vi "Create Downstream View Cavity Spark Scene.vi"(2 "error in (no error)":errorcluster, 3 "Spark Coordinates (cm, rad, cm)":cluster{"r":sgl, "theta":sgl, "z":sgl}) -> (0 "error out":errorcluster, 1 "reference out":refnum<vi>)   [LabVIEW 2013]
uses:
  <vilib>/Utility/miscctls.llb/LV3DPointTypeDef.ctl
  <vilib>/picture/3D Picture Control/Object/Create Object (name).vi
  <vilib>/picture/3D Picture Control/NI_3D Picture Control.lvlib
panel:
  out "Spark Coordinates (cm, rad, rad)":cluster{"rho":dbl, "theta":dbl, "phi":dbl}
  out "Cavity Upstream View":refnum<vi>(3d-picture)
  out "Spark Coordinates (cm, cm, cm)":T1
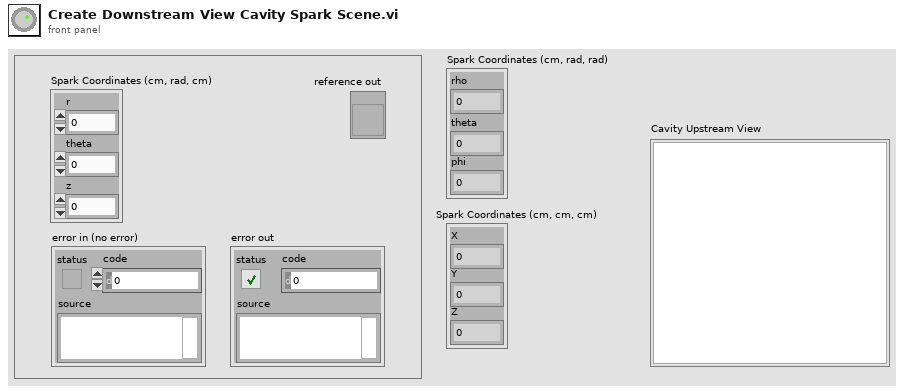
[diagram p1: front panel]
types:
  T1 = typedef "LV3DPointTypeDef.ctl" = cluster{"X":sgl, "Y":sgl, "Z":sgl}
  T2 = cluster{"Red":sgl, "Green":sgl, "Blue":sgl, "Alpha":sgl}
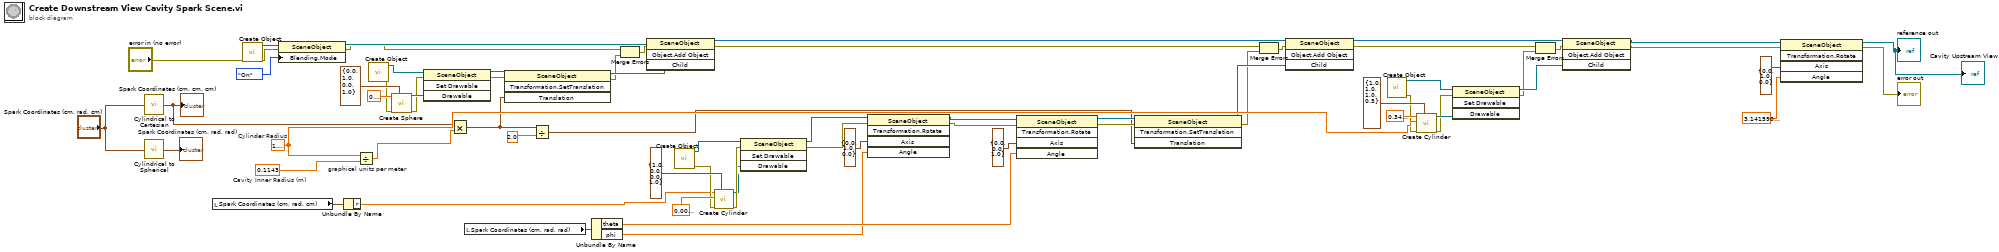
[diagram p0: block diagram]
diagram:
  w52 = 0.1143  # Cavity Inner Radius (m)
  w46 = sgl 1.2  # Cylinder Radius
  n1 = call "Cylindrical to Cartesian.vi"("Cylindrical\nCoordinates"="Spark Coordinates (cm, rad, cm)") -> ("Cartesian\nCoordinates"=w4:cluster{"x":dbl, "y":dbl, "z":dbl})  [unwired: 4 in]
  "Spark Coordinates (cm, cm, cm)" <- w4
  n2 = call "Cylindrical to Spherical.vi"("Cylindrical\nCoordinates"="Spark Coordinates (cm, rad, cm)") -> ("Spherical\nCoordinates"=→"Spark Coordinates (cm, rad, rad)":cluster{"rho":dbl, "theta":dbl, "phi":dbl})  [unwired: 4 in]
  n3 = local read "Spark Coordinates (cm, rad, cm)"() -> (w9:cluster{"r":sgl, "theta":sgl, "z":sgl})
  n4 = call-poly <vilib>:"Create Object.vi"("error in (no error)"="error in (no error)") -> ("error out"=w61:errorcluster, "Scene:New Object"=w62:refnum<vi>)  [unwired: 9 in]
  n5 = property class="SceneObject"(reference=w62, error in=w61, "Blending.Mode"=enum16{"Inherit Value", "Off", "On"}."On" ("Blending:Mode")) -> (reference out=w60:refnum<vi>, error out=w48:errorcluster)
  n6 = Unbundle By Name(w9) -> ("r"=w7:sgl)
  n7 = Divide "graphical units per meter"(x=w46, y=w52) -> (x/y=w22:dbl)
  n8 = call-poly <vilib>:"Create Object.vi"() -> ("error out"=w45:errorcluster, "Scene:New Object"=w58:refnum<vi>)  [unwired: 10 in]
  n9 = call <vilib>:"Create Sphere.vi"("Color"=T2 {"Red"=0.0, "Green"=1.0, "Blue"=0.0, "Alpha"=1.0}, "error in (no error)"=w45, "Radius"=sgl 0.1) -> ("error out"=w44:errorcluster, "New Sphere Refnum"=w64:refnum<vi>)  [unwired: 7 in]
  n10 = invoke class="SceneObject" method="Set Drawable"(reference=w58, error in=w44, "Drawable"=w64) -> (reference out=w55:refnum<vi>, error out=w54:errorcluster)  [unwired: 1 in, 2 out]
  n11 = Multiply(x=w4, y=w22) -> (x*y=w3:cluster{"x":dbl, "y":dbl, "z":dbl})
  n12 = local read "Spark Coordinates (cm, rad, rad)"() -> (w8:cluster{"rho":dbl, "theta":dbl, "phi":dbl})
  n13 = invoke class="SceneObject" method="Transformation.SetTranslation"(reference=w55, error in=w54, "Translation"=w3) -> (reference out=w51:refnum<vi>, error out=w49:errorcluster)  [unwired: 1 in, 2 out]
  n14 = Divide(x=w3, y=sgl 2.0) -> (x/y=w1:cluster{"x":dbl, "y":dbl, "z":dbl})
  n15 = Unbundle By Name(w8) -> ("theta"=w6:dbl, "phi"=w5:dbl)
  n16 = Merge Errors(w48, w49) -> (w50:errorcluster)
  n17 = invoke class="SceneObject" method="Object.Add Object"(reference=w60, error in=w50, "Child"=w51) -> (reference out=w21:refnum<vi>, error out=w20:errorcluster)  [unwired: 1 in, 2 out]
  n18 = call-poly <vilib>:"Create Object.vi"() -> ("error out"=w36:errorcluster, "Scene:New Object"=w38:refnum<vi>)  [unwired: 10 in]
  n19 = call <vilib>:"Create Cylinder.vi"("Color"=T2 {"Red"=1.0, "Green"=0.0, "Blue"=0.0, "Alpha"=1.0}, "error in (no error)"=w36, "Radius"=sgl 0.01, "Height"=w7) -> ("error out"=w35:errorcluster, "New Cylinder Refnum"=w27:refnum<vi>)  [unwired: 6 in]
  n20 = invoke class="SceneObject" method="Set Drawable"(reference=w38, error in=w35, "Drawable"=w27) -> (reference out=w25:refnum<vi>, error out=w24:errorcluster)  [unwired: 1 in, 2 out]
  n21 = invoke class="SceneObject" method="Transformation.Rotate"(reference=w25, error in=w24, "Axis"=T1 {"X"=0.0, "Y"=1.0, "Z"=0.0}, "Angle"=w5) -> (reference out=w31:refnum<vi>, error out=w30:errorcluster)  [unwired: 1 in, 3 out]
  n22 = invoke class="SceneObject" method="Transformation.Rotate"(reference=w31, error in=w30, "Axis"=T1 {"X"=0.0, "Y"=0.0, "Z"=1.0}, "Angle"=w6) -> (reference out=w29:refnum<vi>, error out=w28:errorcluster)  [unwired: 1 in, 3 out]
  n23 = invoke class="SceneObject" method="Transformation.SetTranslation"(reference=w29, error in=w28, "Translation"=w1) -> (reference out=w26:refnum<vi>, error out=w23:errorcluster)  [unwired: 1 in, 2 out]
  n24 = Merge Errors(w20, w23) -> (w34:errorcluster)
  n25 = invoke class="SceneObject" method="Object.Add Object"(reference=w21, error in=w34, "Child"=w26) -> (reference out=w19:refnum<vi>, error out=w18:errorcluster)  [unwired: 1 in, 2 out]
  n26 = call-poly <vilib>:"Create Object.vi"() -> ("error out"=w43:errorcluster, "Scene:New Object"=w57:refnum<vi>)  [unwired: 10 in]
  n27 = call <vilib>:"Create Cylinder.vi"("Color"=T2 {"Red"=1.0, "Green"=1.0, "Blue"=1.0, "Alpha"=0.5}, "error in (no error)"=w43, "Radius"=w46, "Height"=sgl 0.34) -> ("error out"=w42:errorcluster, "New Cylinder Refnum"=w63:refnum<vi>)  [unwired: 6 in]
  n28 = invoke class="SceneObject" method="Set Drawable"(reference=w57, error in=w42, "Drawable"=w63) -> (reference out=w53:refnum<vi>, error out=w41:errorcluster)  [unwired: 1 in, 2 out]
  n29 = Merge Errors(w18, w41) -> (w47:errorcluster)
  n30 = invoke class="SceneObject" method="Object.Add Object"(reference=w19, error in=w47, "Child"=w53) -> (reference out=w13:refnum<vi>, error out=w12:errorcluster)  [unwired: 1 in, 2 out]
  n31 = invoke class="SceneObject" method="Transformation.Rotate"(reference=w13, error in=w12, "Axis"=T1 {"X"=0.0, "Y"=1.0, "Z"=0.0}, "Angle"=sgl 3.14159) -> (reference out=→"reference out" →"Cavity Upstream View":refnum<vi>, error out=→"error out":errorcluster)  [unwired: 1 in, 3 out]
